vi "Facade.vi"(0 "Data In":T5, 2 "Display State In":T3={"Measure ?"=[], "Direction"=[], "Loop ?"={"Start"=0, "Finish"=2}, "Storage Location"=[], "Show Current Location"=FALSE, "Current Location"=0, "Show y=0"=FALSE, "Program"=[], "Index"=0, "Average During Loop ?"=FALSE, "# of Loops"=1, "Loop Control"={0, 2}, "Units"={"Target"="", "Step/Rate"=""}, "Digits"=0, "Significant Figures (F) or DP (T)"=FALSE, "Rate Mode"=FALSE, "Current Y value"=0.0, "Initial Value"=0.0} {"# of Loops" min=1 step=1; "Index" min=0 step=1; "Program"."Step" min=0.001 max=80.0 step=0.001 format="%.2f"; "Program"."Target" format="%.2f"}, 3 "Container State":T4) -> (6 "Data Out":T5, 7 "Display State Out":T3={"Measure ?"=[], "Direction"=[], "Loop ?"={"Start"=0, "Finish"=2}, "Storage Location"=[], "Show Current Location"=FALSE, "Current Location"=0, "Show y=0"=FALSE, "Program"=[], "Index"=0, "Average During Loop ?"=FALSE, "# of Loops"=1, "Loop Control"={0, 2}, "Units"={"Target"="", "Step/Rate"=""}, "Digits"=0, "Significant Figures (F) or DP (T)"=FALSE, "Rate Mode"=FALSE, "Current Y value"=0.0, "Initial Value"=0.0} {"# of Loops" min=1 step=1; "Index" min=0 step=1; "Program"."Step" min=0.001 max=80.0 step=0.001 format="%.2f"; "Program"."Target" format="%.2f"}, 8 "Action":T2)   [LabVIEW 2018, in "Multi Segment Waveform.xctl"]
uses:
  Multi Segment Waveform.xctl
  Data.ctl
  <vilib>/_xctls/Container State.ctl
  State.ctl
  <vilib>/_xctls/Action.ctl
  Support/Type Defs/Formatting Refs.ctl
  <vilib>/_xctls/XControlSupport.lvlib
panel:
  in  "Tab Control":enum32{"Program", "Preview", "Advanced"}(tab)
  out "Mode Label":string="Step"
  in  "Average During Loop ?":bool
  in  "# of Loops":u32=1 min=1 step=1
  in  "Loop ?":cluster{i32, i32}(slide)={0, 2}
  in  "Program":T1(array[cluster]) {"Step" min=0.001 max=80.0 step=0.001 format="%_3p"; "Target" format="%_3p"}
  in  "Index":i32 min=0 step=1
  out "Preview":cluster{dbl[], dbl[]}[](graph)
  in  "Initial Value":dbl
  in  "Save":bool
  in  "Load":bool
  # "Target"
  # "Meas?"
  # "Target"
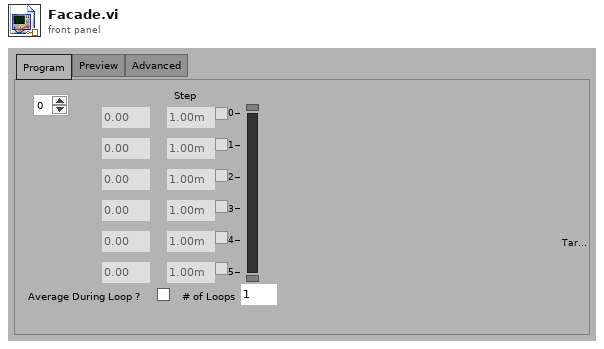
[diagram p1: front panel]
types:
  T1 = cluster{"Target":dbl, "Step":dbl, "Measure ?":bool}[]
  T2 = typedef "XControlSupport.lvlib/Action.ctl" = cluster{"Data Changed?":bool, "State Changed?":bool, "Action Name":string}
  T3 = typedef "Multi Segment Waveform.xctl/State.ctl" = cluster{"Measure ?":bool[], "Direction":bool[], "Loop ?":cluster{"Start":i32, "Finish":i32}, "Storage Location":i32[], "Show Current Location":bool, "Current Location":i32, "Show y=0":bool, "Program":cluster{"Target":dbl, "Step":dbl, "Measure ?":bool}[], "Index":i32, "Average During Loop ?":bool, "# of Loops":u32, "Loop Control":cluster{i32, i32}, "Units":cluster{"Target":string, "Step/Rate":string}, "Digits":i32, "Significant Figures (F) or DP (T)":bool, "Rate Mode":bool, "Current Y value":dbl, "Initial Value":dbl}
  T4 = typedef "XControlSupport.lvlib/Container State.ctl" = cluster{"Indicator?":bool, "Run Mode?":bool, " Refnum":refnum<vi>}
  T5 = typedef "Multi Segment Waveform.xctl/Data.ctl" = waveform(dbl)
  T6 = cluster{"Target":dbl, "Step":dbl, "Measure ?":bool}
  T7 = typedef "Multi Segment Waveform.xctl/Formatting Refs.ctl" = cluster{"Target":refnum<vi>, "Step":refnum<vi>, "Mode Label":refnum<vi>, "Initial Value Ref":refnum<vi>, "Program Ref":refnum<vi>}
  T8 = typedef "LVRectTypeDef.ctl" = cluster{"Left":i16, "Top":i16, "Right":i16, "Bottom":i16}
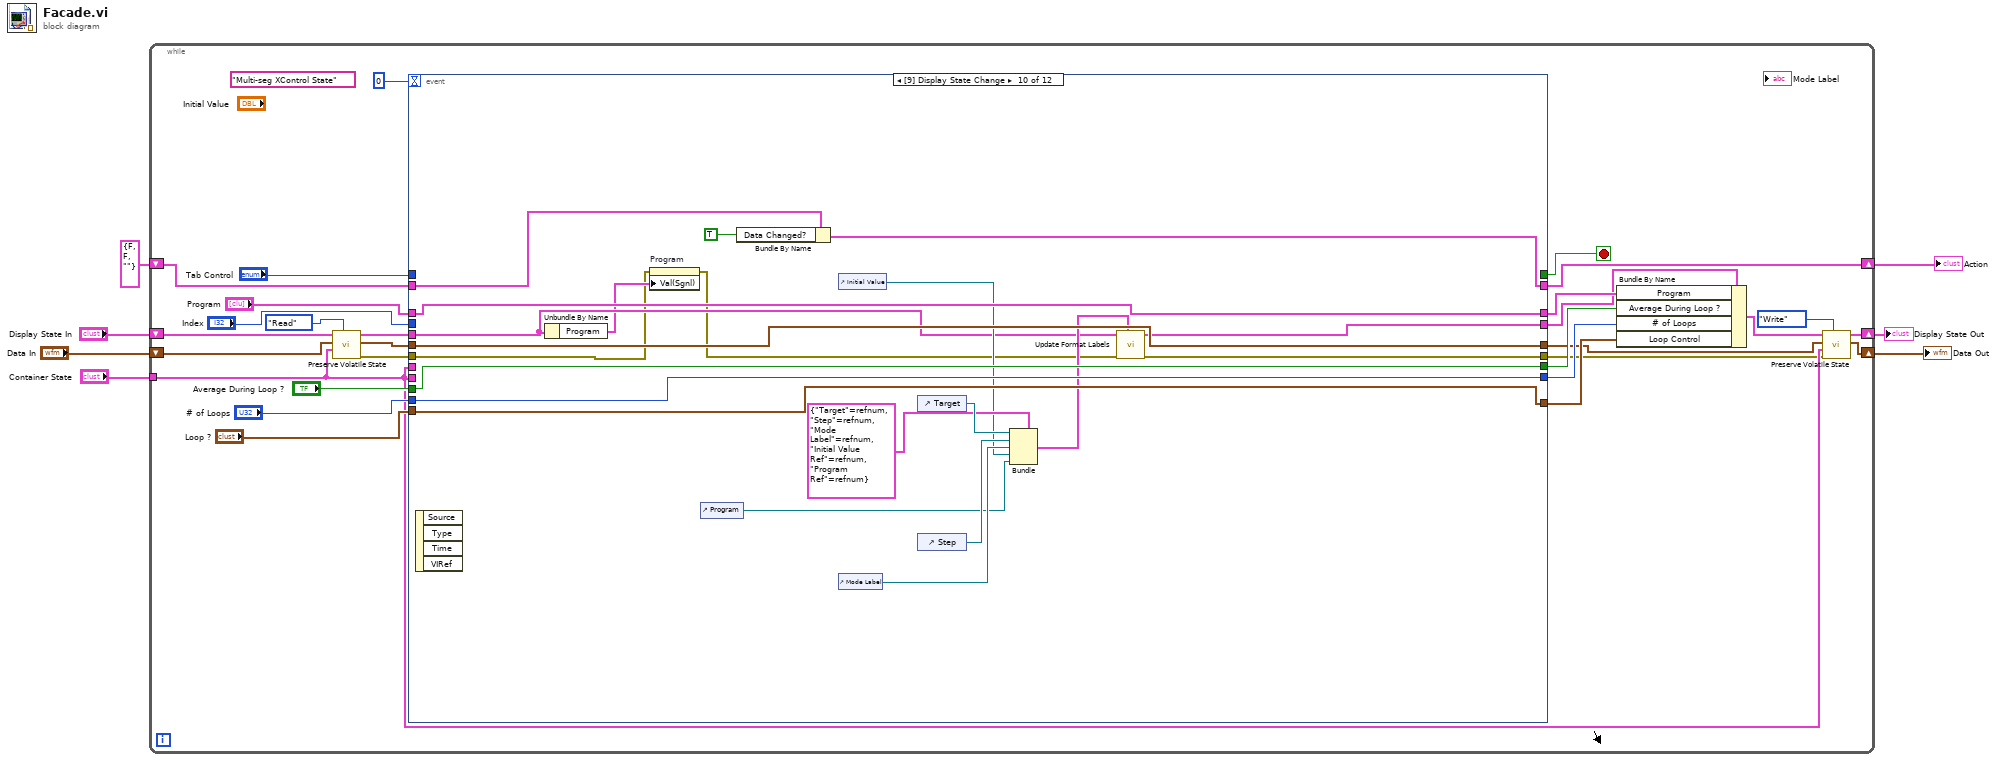
[diagram p0: block diagram]
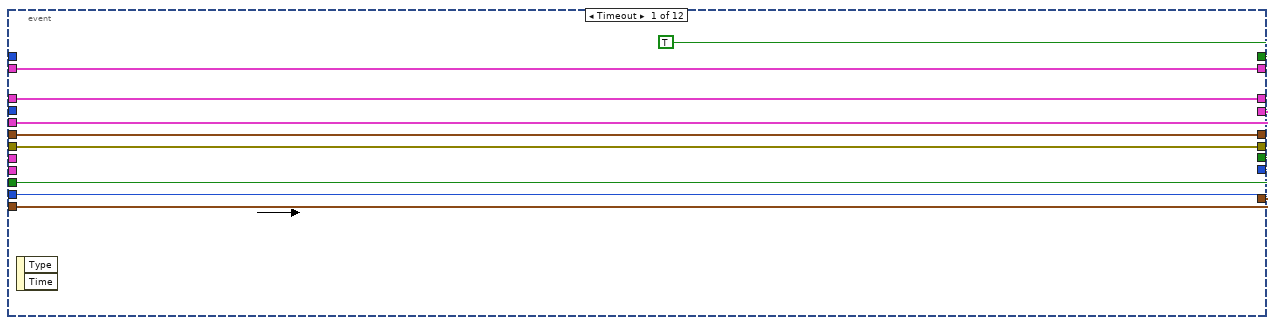
[diagram p2: hidden frame]
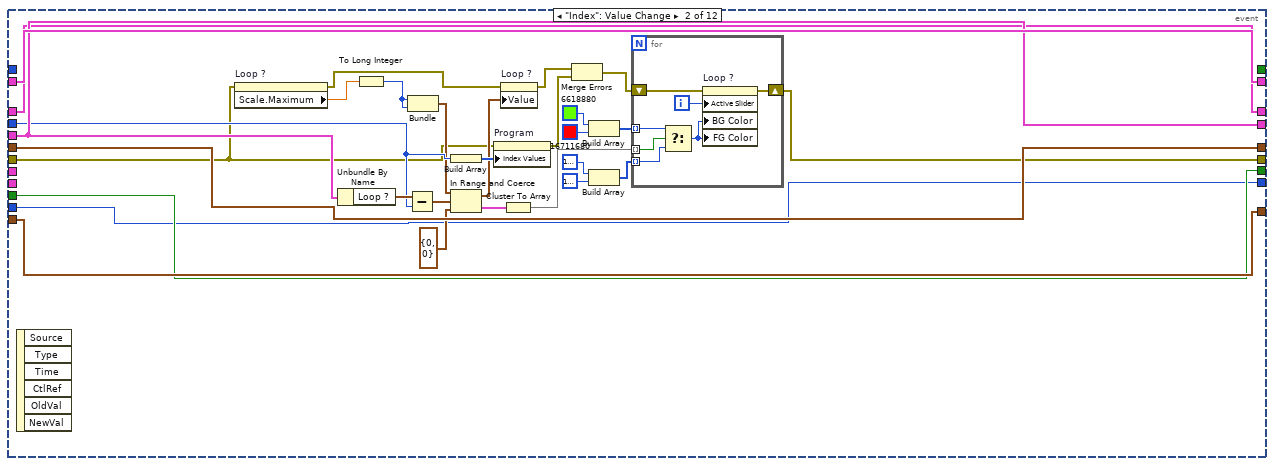
[diagram p3: hidden frame]
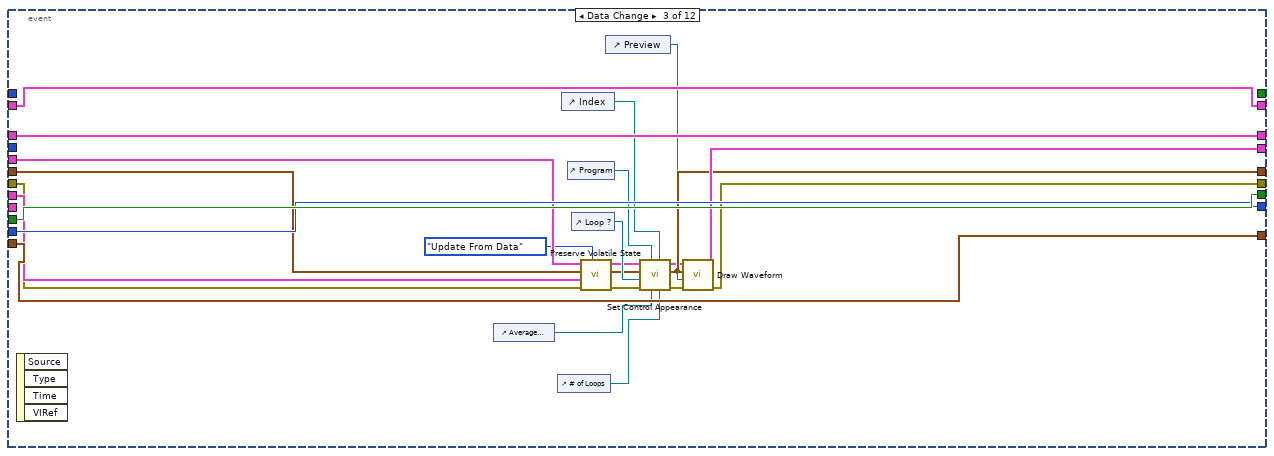
[diagram p4: hidden frame]
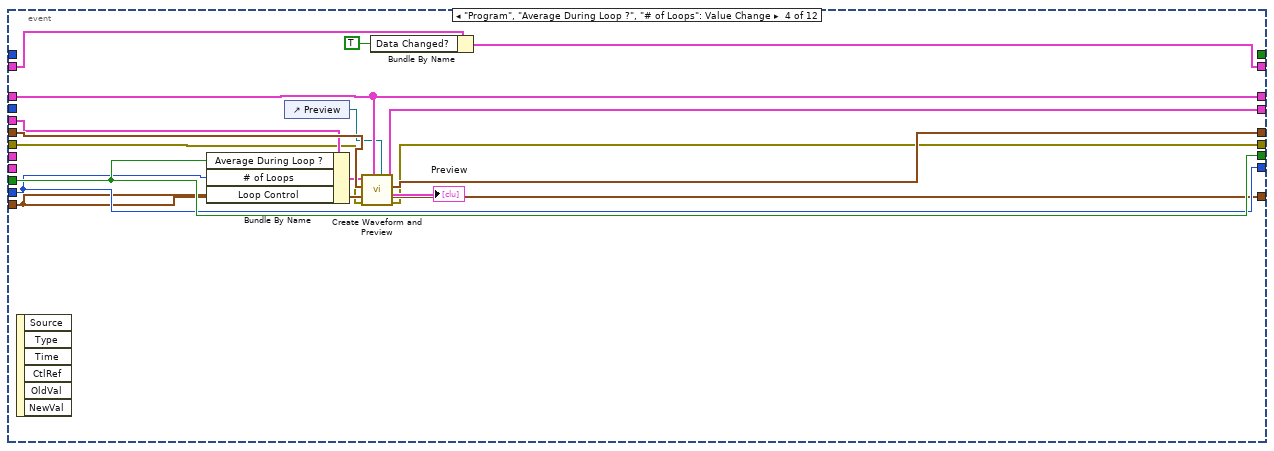
[diagram p5: hidden frame]
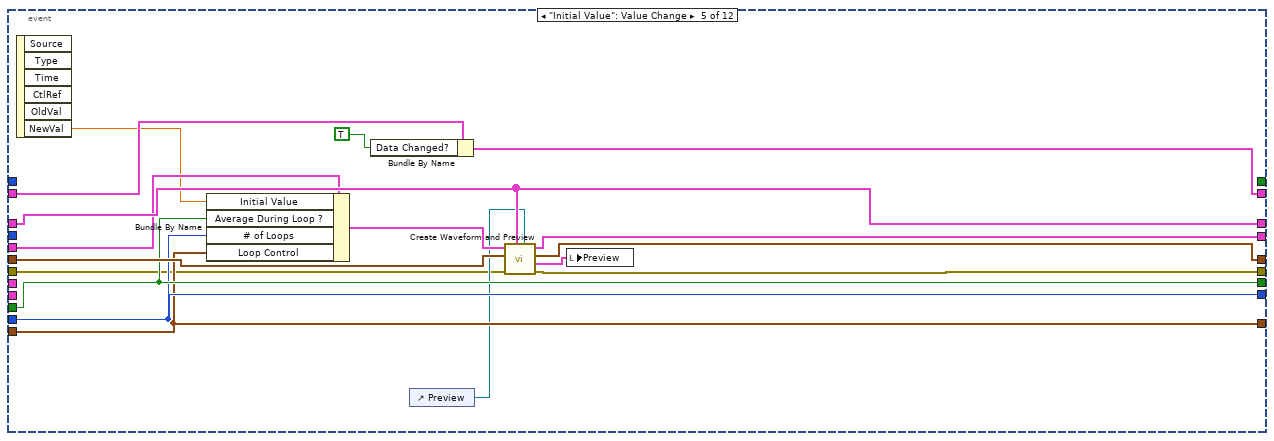
[diagram p6: hidden frame]
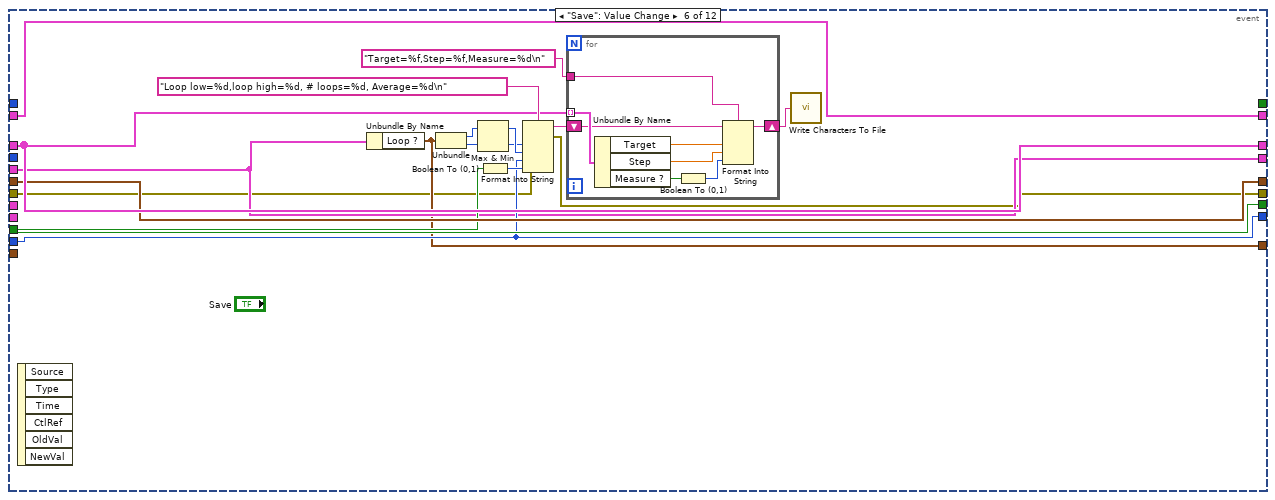
[diagram p7: hidden frame]
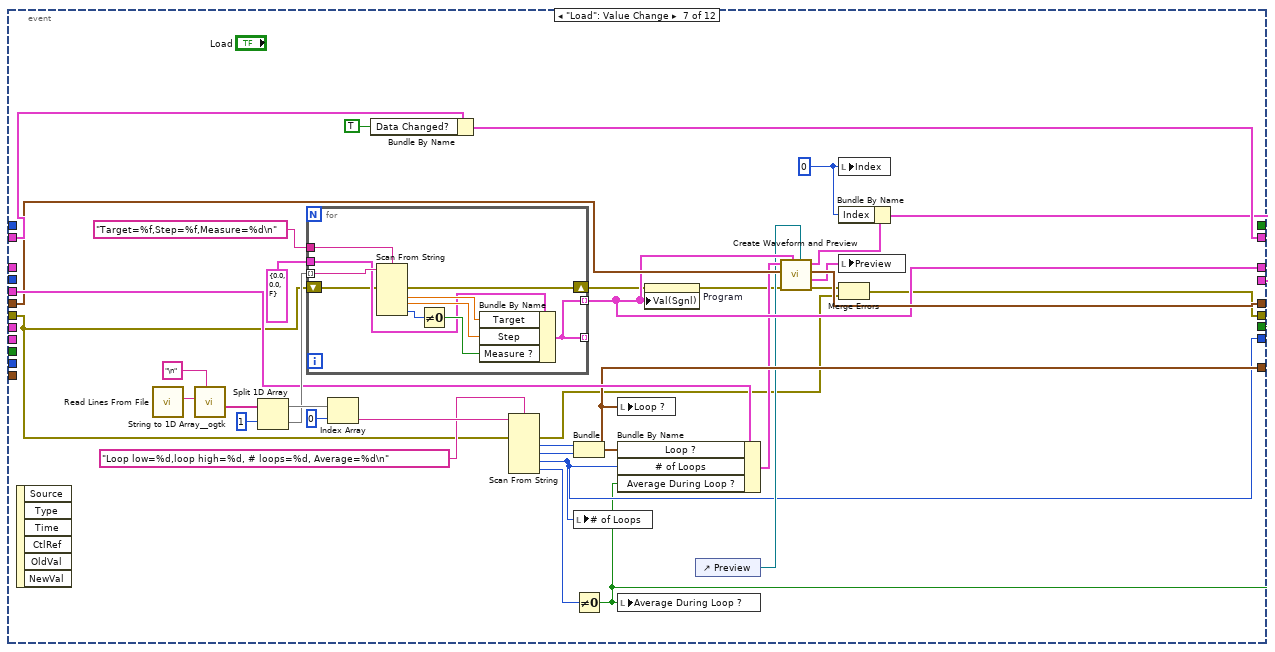
[diagram p8: hidden frame]
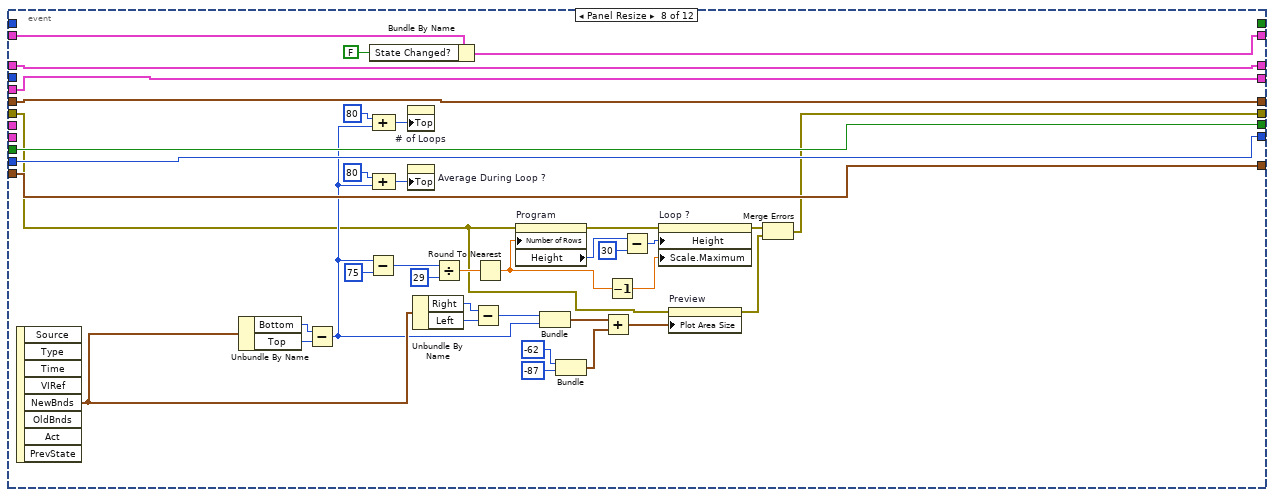
[diagram p9: hidden frame]
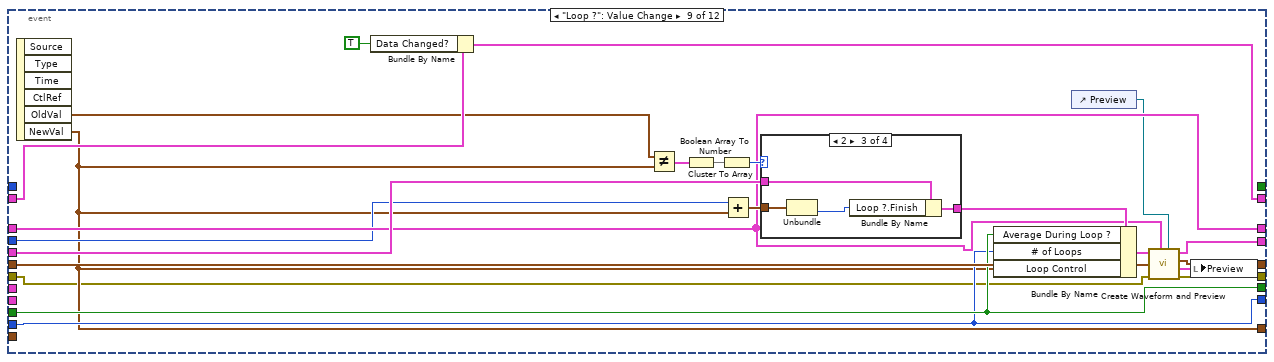
[diagram p10: hidden frame]
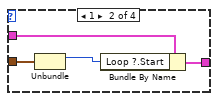
[diagram p12: hidden frame]
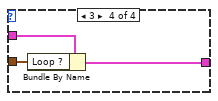
[diagram p13: hidden frame]
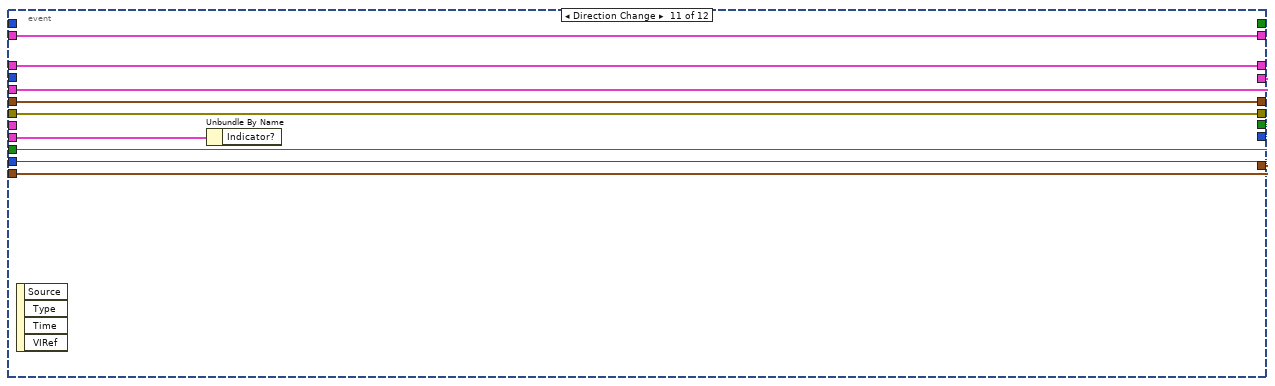
[diagram p14: hidden frame]
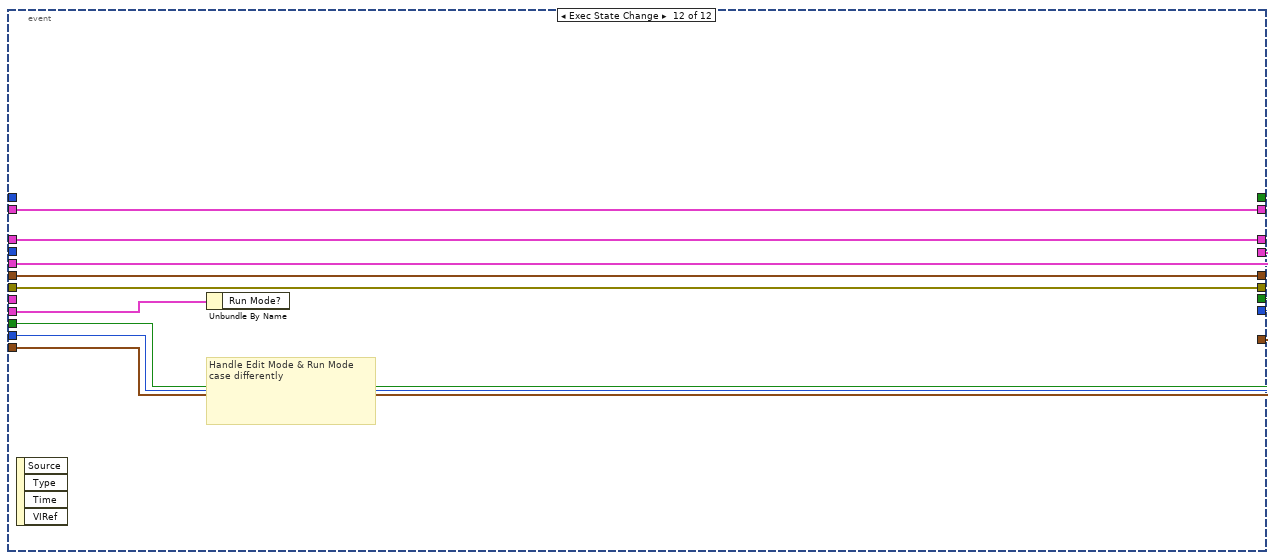
[diagram p15: hidden frame]
diagram:
  n1 = while {
    shift-right: [w21] -> w4
    shift-left: "Display State In" -> [w19]
    tunnel: "Container State" -> [w10]
    shift-right: [w11] -> w7
    shift-left: "Data In" -> [w15]
    shift-right: [w32] -> w2
    shift-left: T2 {"Data Changed?"=FALSE, "State Changed?"=FALSE, "Action Name"=""} ("Action") -> [w33]
    stop <- w35 stop-if-true
    (unwired) "Multi-seg XControl State" ("name")
    n2 = call "Preserve Volatile State.vi"("Operation"=enum16{"Read", "Write", "Update From Data"}."Read", "Container State"=w10, "Waveform"=w15, "Waveform State In"=w19) -> ("error out"=w9:errorcluster, "Waveform Out"=w14:T5, "Waveform State Out"=w18:T3)  [unwired: 1 in, 4 out]
    n3 = event shown="[9] Display State Change" {
      selector: _ -> [_ _ _ _ _ _ _ _ _ _ _ _]
      dyn-events: _ -> [_ _ _ _ _ _ _ _ _ _ _ _]
      timeout: 0 -> [_ _ _ _ _ _ _ _ _ _ _ _]
      tunnel: w18 -> [w42 w71 w90 w114 w131 w143 w190 w245 w272 w288 w313 w322]
      tunnel: [w42 w71 w100 w120 w137 w143 w178 w245 w260 w297 w313 w322] -> w17
      tunnel: [TRUE _ _ _ _ _ _ _ _ _ _ _] -> w35
      tunnel: w10 -> [_ _ _ _ _ _ _ _ _ _ w314 w323]
      tunnel: w14 -> [w41 w73 w86 w121 w138 w147 w187 w249 w263 w304 w312 w321]
      tunnel: [w41 w73 w99 w115 w132 w147 w186 w249 w262 w304 w312 w321] -> w12
      tunnel: [w43 w74 w105 w117 w134 w146 w180 w247 w270 w299 w311 w320] -> w32
      tunnel: w33 -> [w43 w74 w105 w118 w135 w146 w189 w248 w271 w305 w311 w320]
      tunnel: "# of Loops" -> [w37 w51 w101 w109 w128 w144 _ w229 w253 w300 w307 w316]
      tunnel: "Loop ?" -> [w39 w53 w103 w108 w127 _ _ w231 _ w302 w309 w318]
      tunnel: "Program" -> [w40 w54 w104 w119 w136 w148 _ w232 w258 w303 w310 w319]
      tunnel: "Average During Loop ?" -> [w38 w52 w102 w110 w129 w145 _ w230 w254 w301 w308 w317]
      tunnel: "Index" -> [_ w68 _ _ _ _ _ _ w256 _ _ _]
      tunnel: [w40 w54 w104 w119 w136 w148 w185 w232 w258 w303 w310 w319] -> w30
      tunnel: [w39 w53 w103 w108 w127 w142 w188 w231 w252 w302 w309 w318] -> w28
      tunnel: [w38 w52 w102 w110 w129 w145 w171 w230 w254 w301 w308 w317] -> w26
      tunnel: [w37 w51 w101 w109 w128 w144 w172 w229 w253 w300 w307 w316] -> w24
      tunnel: "Tab Control" -> [_ _ _ _ _ _ _ _ _ _ _ _]
      tunnel: w10 -> [_ _ w84 _ _ _ _ _ _ _ _ _]
      tunnel: w9 -> [w36 w48 w83 w106 w123 w140 w169 w215 w250 w286 w306 w315]
      tunnel: [w36 w50 w82 w107 w122 w139 w166 w212 w251 w290 w306 w315] -> w8
      event Timeout {
        n4 = event-data() -> ()  [unwired: 3 out]
      }
      event "Index": Value Change {
        n5 = event-data() -> ()  [unwired: 7 out]
        n6 = property on="Loop ?" class="Slide (strict)"(error in=w48) -> (error out=w49:errorcluster, "Scale.Maximum"=w57:dbl)  [unwired: 1 in, 1 out]
        n7 = Unbundle By Name(w71) -> ("Loop ?"=w70:cluster{"Start":i32, "Finish":i32})
        n8 = To Long Integer(number=w57) -> (32bit integer=w56:i32)
        n9 = Subtract(x=w70, y=w68) -> (x-y=w69:cluster{"Start":i32, "Finish":i32})
        n10 = Bundle(w56, w56) -> (w55:cluster{i32, i32})  [unwired: 1 out]
        n11 = Build Array(w68) -> (w72:i32[])
        n12 = In Range and Coerce(upper limit=w55, x=w69, lower limit=cluster{i32, i32} {0, 0}) -> (coerced(x)=w67:cluster{"Start":i32, "Finish":i32}, In Range?=w65:cluster{"Start":bool, "Finish":bool})
        n13 = property on="Program" class="Arr (strict)"(error in=w48, "Index Values"=w72) -> (error out=w45:errorcluster)  [unwired: 1 in, 1 out]
        n14 = property on="Loop ?" class="Slide (strict)"(error in=w49, "Value"=w67) -> (error out=w47:errorcluster)  [unwired: 1 in, 1 out]
        n15 = Cluster To Array(cluster=w65) -> (array=w64:bool[])
        n16 = Merge Errors(w47, w45) -> (w46:errorcluster)
        n17 = Build Array(u32 6618880, u32 16711680) -> (w61:u32[])
        n18 = Build Array(u32 16777216, u32 16777216) -> (w58:u32[])
        n19 = for {
          tunnel: w64 -> [w81] mode=indexing
          tunnel: w61 -> [w79] mode=indexing
          tunnel: w58 -> [w78] mode=indexing
          shift-right: [w75] -> w50
          shift-left: w46 -> [w76]
          i -> [w80]
          n20 = Select(t=w79, s=w81, f=w78) -> (s? t:f=w77:u32)
          n21 = property on="Loop ?" class="Slide (strict)"(error in=w76, "Active Slider"=w80, "BG Color"=w77, "FG Color"=w77) -> (error out=w75:errorcluster)  [unwired: 1 in, 1 out]
        }
      }
      event Data Change {
        n22 = event-data() -> ()  [unwired: 5 out]
        n23 = control-ref of="Average During Loop ?"() -> (w95:refnum<vi>)
        n24 = control-ref of="# of Loops"() -> (w94:refnum<vi>)
        n25 = control-ref of="Index"() -> (w96:refnum<vi>)
        n26 = control-ref of="Program"() -> (w97:refnum<vi>)
        n27 = control-ref of="Loop ?"() -> (w93:refnum<vi>)
        n28 = call "Preserve Volatile State.vi"("Operation"=enum16{"Read", "Write", "Update From Data"}."Update From Data", "error in (no error)"=w83, "Container State"=w84, "Waveform"=w86, "Waveform State In"=w90) -> ("error out"=w87:errorcluster, "Waveform Out"=w85:T5, "Waveform State Out"=w89:T3)  [unwired: 4 out]
        n29 = control-ref of="Preview"() -> (w91:refnum<vi>)
        n30 = call "Set Control Appearance.vi"("DigNum Refnum 2"=w94, "DigNum Refnum"=w96, "Bool Refnum"=w95, "Arr Refnum"=w97, "error in (no error)"=w87, "Slide Refnum"=w93, "Data In"=w85, "Display State In"=w89) -> ("error out"=w98:errorcluster, "Data Out"=w99:T5, "Display State Out"=w92:T3)  [unwired: 1 out]
        n31 = call "Draw Waveform.vi"("Error"=w98, "Ref"=w91, "Data"=w99, "Display State"=w92) -> ("Error Out"=w82:errorcluster, "Display State Out"=w100:T3)  [unwired: 1 in, 5 out]
      }
      event "Program", "Average During Loop ?", "# of Loops": Value Change {
        n32 = event-data() -> ()  [unwired: 7 out]
        n33 = Bundle By Name(cluster=w114, "Average During Loop ?"=w110, "# of Loops"=w109, "Loop Control"=w108) -> (w111:T3)
        n34 = control-ref of="Preview"() -> (w113:refnum<vi>)
        n35 = call "Create Waveform and Preview.vi"("XYGraph Refnum"=w113, "Program"=w119, "error in (no error)"=w106, "Waveform In"=w121, "Display State In"=w111) -> ("error out"=w107:errorcluster, "Preview Graph"=→"Preview":cluster{dbl[], dbl[]}[], "Waveform Out"=w115:T5, "State Out"=w120:T3)  [unwired: 2 in, 1 out]
        n36 = Bundle By Name(cluster=w118, "Data Changed?"=TRUE) -> (w117:T2)
      }
      event "Initial Value": Value Change {
        n37 = event-data() -> ("NewVal"=w125:dbl)  [unwired: 6 out]
        n38 = Bundle By Name(cluster=w131, "Initial Value"=w125, "Average During Loop ?"=w129, "# of Loops"=w128, "Loop Control"=w127) -> (w130:T3)
        n39 = Bundle By Name(cluster=w135, "Data Changed?"=TRUE) -> (w134:T2)
        n40 = control-ref of="Preview"() -> (w124:refnum<vi>)
        n41 = call "Create Waveform and Preview.vi"("XYGraph Refnum"=w124, "Program"=w136, "error in (no error)"=w123, "Waveform In"=w138, "Display State In"=w130) -> ("error out"=w122:errorcluster, "Preview Graph"=w126:cluster{dbl[], dbl[]}[], "Waveform Out"=w132:T5, "State Out"=w137:T3)  [unwired: 2 in, 1 out]
        n42 = local write "Preview"(w126) -> ()
      }
      event "Save": Value Change {
        n43 = event-data() -> ()  [unwired: 7 out]
        n44 = Unbundle By Name(w143) -> ("Loop ?"=w142:cluster{"Start":i32, "Finish":i32})
        n45 = Unbundle(w142) -> ("Start"=w149:i32, "Finish"=w150:i32)
        n46 = Max & Min(x=w149, y=w150) -> (max(x,y)=w153:i32, min(x,y)=w152:i32)
        n47 = Boolean To (0,1)(Boolean=w145) -> (0, 1=w154:i16)
        n48 = Format Into String(format string="Loop low=%d,loop high=%d, # loops=%d, Average=%d\n", error in=w140, w152, w153, w144, w154) -> (resulting string=w155:string, error out=w139:errorcluster)  [unwired: 1 in]
        n49 = for {
          tunnel: w148 -> [w164] mode=indexing
          shift-right: [w158] -> w156
          shift-left: w155 -> [w159]
          tunnel: "Target=%f,Step=%f,Measure=%d\n" -> [w157]
          n50 = Unbundle By Name(w164) -> ("Target"=w160:dbl, "Step"=w162:dbl, "Measure ?"=w163:bool)
          n51 = Boolean To (0,1)(Boolean=w163) -> (0, 1=w161:i16)
          n52 = Format Into String(format string=w157, initial string=w159, w160, w162, w161) -> (resulting string=w158:string)  [unwired: 1 in, 1 out]
        }
        n53 = call <vilib>:"Write Characters To File.vi"("character string"=w156) -> ()  [unwired: 2 in, 3 out]
      }
      event "Load": Value Change {
        w177 = 0 ("Index")
        n54 = event-data() -> ()  [unwired: 7 out]
        n55 = call <vilib>:"Read Lines From File.vi"() -> ("line string"=w174:string)  [unwired: 2 in, 7 out]
        n56 = call <userlib>:"String to 1D Array__ogtk.vi"("delimiter (Tab)"="\n", "string"=w174) -> ("Array of Strings"=w173:string[])  [unwired: 1 in, 8 out]
        n57 = Split 1D Array(array=w173, index=1) -> (first subarray=w195:string[], second subarray=w193:string[])
        n58 = for {
          tunnel: w193 -> [w210] mode=indexing
          tunnel: [w204] -> _ mode=indexing
          tunnel: [w204] -> w185 mode=indexing
          tunnel: T6 {"Target"=0.0, "Step"=0.0, "Measure ?"=FALSE} ("Cluster") -> [w205]
          tunnel: "Target=%f,Step=%f,Measure=%d\n" -> [w203]
          shift-right: [w201] -> w170
          shift-left: w169 -> [w202]
          n59 = Scan From String(format string=w203, input string=w210, error in=w202) -> (error out=w201:errorcluster, output 1=w206:dbl, output 2=w207:dbl, output 3=w209:i32)  [unwired: 1 in, 5 out]
          n60 = Not Equal To 0?(x=w209) -> (x != 0?=w208:bool)
          n61 = Bundle By Name(cluster=w205, "Target"=w206, "Step"=w207, "Measure ?"=w208) -> (w204:T6)
        }
        n62 = Index Array(array=w195, index=0 ("Index")) -> (element=w197:string)
        n63 = Bundle By Name(cluster=w189, "Data Changed?"=TRUE) -> (w180:T2)
        n64 = Scan From String(format string="Loop low=%d,loop high=%d, # loops=%d, Average=%d\n", input string=w197, error in=w169) -> (error out=w165:errorcluster, output 1=w198:i32, output 2=w199:i32, output 3=w172:i32, output 4=w200:i32)  [unwired: 1 in, 6 out]
        n65 = Bundle(w198, w199) -> (w188:cluster{i32, i32})  [unwired: 1 out]
        n66 = local write "# of Loops"(w172) -> ()
        n67 = Not Equal To 0?(x=w200) -> (x != 0?=w171:bool)
        n68 = local write "Loop ?"(w188) -> ()
        n69 = Bundle By Name(cluster=w190, "Loop ?"=w188, "# of Loops"=w172, "Average During Loop ?"=w171) -> (w184:T3)
        n70 = local write "Average During Loop ?"(w171) -> ()
        n71 = property on="Program" class="Arr (strict)"(error in=w170, "Val(Sgnl)"=w185) -> (error out=w168:errorcluster)  [unwired: 1 in, 1 out]
        n72 = control-ref of="Preview"() -> (w181:refnum<vi>)
        n73 = call "Create Waveform and Preview.vi"("XYGraph Refnum"=w181, "Program"=w185, "error in (no error)"=w168, "Waveform In"=w187, "Display State In"=w184) -> ("error out"=w167:errorcluster, "Preview Graph"=w182:cluster{dbl[], dbl[]}[], "Waveform Out"=w186:T5, "State Out"=w183:T3)  [unwired: 2 in, 1 out]
        n74 = local write "Index"(w177) -> ()
        n75 = Bundle By Name(cluster=w183, "Index"=w177) -> (w178:T3)
        n76 = local write "Preview"(w182) -> ()
        n77 = Merge Errors(w167, w165) -> (w166:errorcluster)
      }
      event Panel Resize {
        n78 = event-data() -> ("NewBnds"=w228:T8)  [unwired: 8 out]
        n79 = Unbundle By Name(w228) -> ("Bottom"=w236:i16, "Top"=w235:i16)
        n80 = Subtract(x=w236, y=w235) -> (x-y=w220:i16)
        n81 = Subtract(x=w220, y=i16 75) -> (x-y=w233:i16)
        n82 = Bundle By Name(cluster=w248, "State Changed?"=FALSE) -> (w247:T2)
        n83 = Compound Arithmetic op=ADD(i16 80 ("value"), w220) -> (w224:i16)
        n84 = Compound Arithmetic op=ADD(i16 80 ("value"), w220) -> (w223:i16)
        n85 = property on="# of Loops" class="DigNum (strict)"("Top"=w224) -> ()  [unwired: 2 in, 2 out]
        n86 = property on="Average During Loop ?" class="Bool (strict)"("Top"=w223) -> ()  [unwired: 2 in, 2 out]
        n87 = Unbundle By Name(w228) -> ("Right"=w227:i16, "Left"=w226:i16)
        n88 = Divide(x=w233, y=u32 29) -> (x/y=w239:dbl)
        n89 = Subtract(x=w227, y=w226) -> (x-y=w221:i16)
        n90 = Round To Nearest(number=w239) -> (nearest integer value=w241:dbl)
        n91 = property on="Program" class="Arr (strict)"(error in=w215, "Number of Rows"=w241) -> (error out=w214:errorcluster, "Height"=w244:u32)  [unwired: 1 in, 1 out]
        n92 = Bundle(w221, w220) -> (w219:cluster{i16, i16})  [unwired: 1 out]
        n93 = Bundle("value"=i16 -62, "value"=i16 -87) -> (w218:cluster{"value":i16, "value":i16})  [unwired: 1 out]
        n94 = Add(x=w219, y=w218) -> (x+y=w238:cluster{i16, i16})
        n95 = Decrement(x=w241) -> (x-1=w240:dbl)
        n96 = Subtract(x=w244, y=u32 30) -> (x-y=w242:u32)
        n97 = property on="Loop ?" class="Slide (strict)"(error in=w214, "Height"=w242, "Scale.Maximum"=w240) -> (error out=w213:errorcluster)  [unwired: 1 in, 1 out]
        n98 = property on="Preview" class="XYGraph (strict)"(error in=w215, "Plot Area Size"=w238) -> (error out=w211:errorcluster)  [unwired: 1 in, 1 out]
        n99 = Merge Errors(w213, w211) -> (w212:errorcluster)
      }
      event "Loop ?": Value Change {
        n100 = event-data() -> ("OldVal"=w268:cluster{i32, i32}, "NewVal"=w252:cluster{i32, i32})  [unwired: 5 out]
        n101 = Bundle By Name(cluster=w271, "Data Changed?"=TRUE ("State Changed?")) -> (w270:T2)
        n102 = Not Equal?(x=w268, y=w252) -> (x != y?=w267:cluster{bool, bool})
        n103 = Cluster To Array(cluster=w267) -> (array=w266:bool[])
        n104 = Boolean Array To Number(Boolean array=w266) -> (number=w265:u32)
        n105 = Add(x=w256, y=w252) -> (x+y=w264:cluster{i32, i32})
        n106 = case shown="2" w265 {
          tunnel: w272 -> [w273 w277 w281 w284]
          tunnel: [w273 w276 w280 w283] -> w259
          tunnel: w264 -> [_ w275 w279 w282]
          frame 0, Default {
          }
          frame 1 {
            n107 = Unbundle(w275) -> (w274:i32)  [unwired: 1 out]
            n108 = Bundle By Name(cluster=w277, "Loop ?.Start"=w274) -> (w276:T3)
          }
          frame 2 {
            n109 = Unbundle(w279) -> (w278:i32)  [unwired: 1 out]
            n110 = Bundle By Name(cluster=w281, "Loop ?.Finish"=w278) -> (w280:T3)
          }
          frame 3 {
            n111 = Bundle By Name(cluster=w284, "Loop ?"=w282) -> (w283:T3)
          }
        }
        n112 = Bundle By Name(cluster=w259, "Average During Loop ?"=w254, "# of Loops"=w253, "Loop Control"=w252) -> (w255:T3)
        n113 = control-ref of="Preview"() -> (w257:refnum<vi>)
        n114 = call "Create Waveform and Preview.vi"("XYGraph Refnum"=w257, "Program"=w258, "error in (no error)"=w250, "Waveform In"=w263, "Display State In"=w255) -> ("error out"=w251:errorcluster, "Preview Graph"=w261:cluster{dbl[], dbl[]}[], "Waveform Out"=w262:T5, "State Out"=w260:T3)  [unwired: 2 in, 1 out]
        n115 = local write "Preview"(w261) -> ()
      }
      event Display State Change {
        n116 = event-data() -> ()  [unwired: 5 out]
        n117 = Unbundle By Name(w288) -> ("Program"=w287:T1)
        n118 = property on="Program" class="Arr (strict)"(error in=w286, "Val(Sgnl)"=w287) -> (error out=w285:errorcluster)  [unwired: 1 in, 1 out]
        n119 = control-ref of="Program"() -> (w289:refnum<vi>)
        n120 = Bundle By Name(cluster=w305, "Data Changed?"=TRUE) -> (w299:T2)
        n121 = control-ref of="Initial Value"() -> (w291:refnum<vi>)
        n122 = control-ref of="Mode Label"() -> (w294:refnum<vi>)
        n123 = control-ref of="Target"() -> (w296:refnum<vi>)
        n124 = control-ref of="Step"() -> (w295:refnum<vi>)
        n125 = Bundle(cluster=T7 {"Target"=refnum, "Step"=refnum, "Mode Label"=refnum, "Initial Value Ref"=refnum, "Program Ref"=refnum} ("Format Cluster"), "Target"=w296, "Step"=w295, "Mode Label"=w294, "Initial Value Ref"=w291, "Program Ref"=w289) -> (w293:T7)
        n126 = call "Update Format Labels.vi"("Format Cluster"=w293, "error in (no error)"=w285, "State In"=w288) -> ("error out"=w290:errorcluster, "State Out"=w297:T3)  [unwired: 7 out]
      }
      event Direction Change {
        n127 = event-data() -> ()  [unwired: 5 out]
        n128 = Unbundle By Name(w314) -> ()  [unwired: 1 out]
      }
      event Exec State Change {
        # "Handle Edit Mode & Run Mode\ncase differently"
        n129 = event-data() -> ()  [unwired: 5 out]
        n130 = Unbundle By Name(w323) -> ()  [unwired: 1 out]
      }
    }
    n131 = Bundle By Name(cluster=w17, "Program"=w30, "Average During Loop ?"=w26, "# of Loops"=w24, "Loop Control"=w28) -> (w13:T3)
    n132 = call "Preserve Volatile State.vi"("Operation"=enum16{"Read", "Write"}."Write", "error in (no error)"=w8, "Container State"=w10, "Waveform"=w12, "Waveform State In"=w13) -> ("Waveform Out"=w11:T5, "Waveform State Out"=w21:T3)  [unwired: 5 out]
  }
  "Display State Out" <- w4
  "Data Out" <- w7
  "Action" <- w2
